vi "List-All-Label's.vi"(8 "error in (no error)":errorcluster, 11 "Quick-GUI-Update in":refnum<class "Quick-GUI-Update.lvclass">) -> (0 "error out":errorcluster, 1 "Label's List":string[][](array[string]), 3 "Quick-GUI-Update out":refnum<class "Quick-GUI-Update.lvclass">)   [LabVIEW 2020, in "Quick-GUI-Update.lvclass"]
uses:
  Quick-GUI-Update.lvclass
  Quick-GUI-Update.lvclass/Quick-GUI-Update.ctl
  Ctrl Reference's/Ctrl Reference's.lvclass
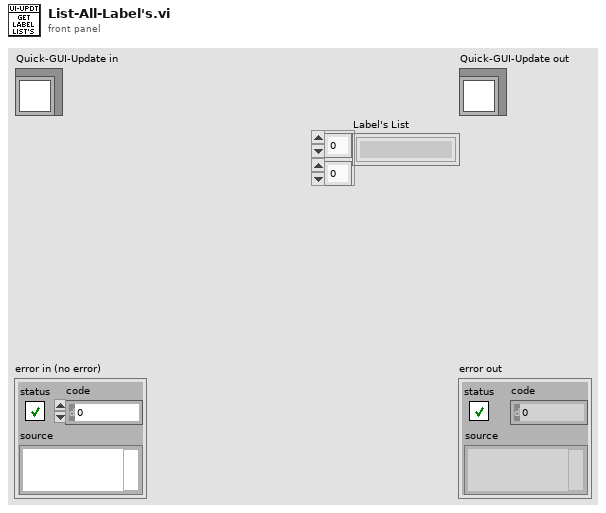
[diagram p1: front panel]
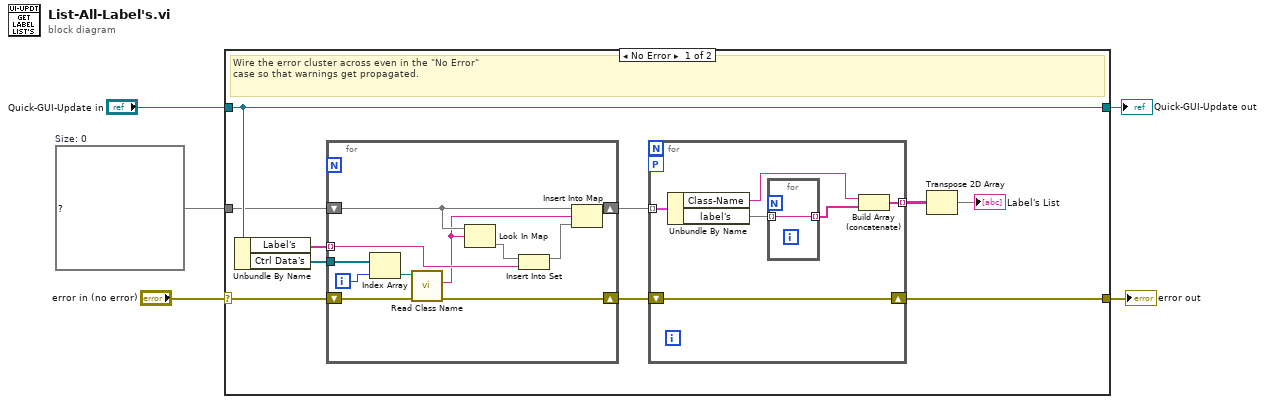
[diagram p0: block diagram]
diagram:
  w1 = map{string, set{string}} {}  # Size: 0
  n1 = case shown="No Error" "error in (no error)" {
    selector: "error in (no error)" -> [w14 w35]
    tunnel: [w8 w35] -> w4
    tunnel: [w15 w34] -> w2
    tunnel: "Quick-GUI-Update in" -> [w15 w34]
    tunnel: w1 -> [w13 _]
    frame No Error {
      # "Wire the error cluster across even in the \"No Error\"\ncase so that warnings get propagated."
      n2 = Unbundle By Name(w15) -> ("Label's"=w7:string[], "Ctrl Data's"=w6:refnum<class "Ctrl Reference's.lvclass">[])
      n3 = for {
        shift-right: [w32] -> w10
        shift-left: w13 -> [w33]
        shift-right: [w23] -> w9
        shift-left: w14 -> [w25]
        tunnel: w7 -> [w29] mode=indexing
        tunnel: w6 -> [w28]
        i -> [w27]
        n4 = Index Array(array=w28, index=w27) -> (element=w26:refnum<class "Ctrl Reference's.lvclass">)
        n5 = call-dynamic "Read Class Name.vi"("error in (no error)"=w25, "Ctrl Reference's in"=w26) -> ("error out"=w23:errorcluster, "Class Name"=w24:string)  [unwired: 7 in, 1 out]
        n6 = Look In Map(map=w33, key=w24) -> (value=w31:set{string})  [unwired: 1 in, 1 out]
        n7 = Insert Into Set(10:w29, 11:w31) -> (3:w30:set{string})  [unwired: 1 out]
        n8 = Insert Into Map(map in=w33, key=w24, value=w30) -> (map out=w32:map{string, set{string}})  [unwired: 2 out]
      }
      n9 = for {
        tunnel: w10 -> [w21] mode=indexing
        tunnel: [w17] -> w12 mode=indexing
        shift-right: [w16] -> w8
        shift-left: w9 -> [w16]
        workers-P: _ -> [_]
        n10 = Unbundle By Name(w21) -> ("Class-Name"=w18:string, "label's"=w20:set{string})
        n11 = for {
          tunnel: w20 -> [w22] mode=indexing
          tunnel: [w22] -> w19 mode=indexing
        }
        n12 = Build Array (concatenate)(w18, w19) -> (w17:string[])
      }
      n13 = Transpose 2D Array(2D array=w12) -> (transposed array=→"Label's List":string[][])
    }
    frame Error {
    }
  }
  "error out" <- w4
  "Quick-GUI-Update out" <- w2
